vi "Get Request Type.vi"(8 "error in (no error)":errorcluster, 11 "GetStreamStatus in":refnum<class "GetStreamStatus.lvclass">) -> (0 "error out":errorcluster, 2 "Request Type":string, 3 "GetStreamStatus out":refnum<class "GetStreamStatus.lvclass">)   [LabVIEW 2022 SP3, in "obs-websocket-lv.lvlib" / "GetStreamStatus.lvclass"]
uses:
  GetStreamStatus.lvclass
  GetStreamStatus.lvclass/GetStreamStatus.ctl
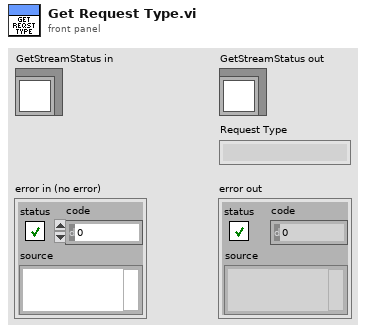
[diagram p1: front panel]
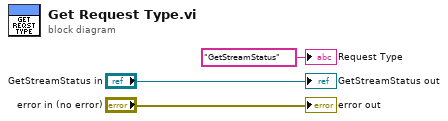
[diagram p0: block diagram]
diagram:
  "error out" <- "error in (no error)"
  "GetStreamStatus out" <- "GetStreamStatus in"
  "Request Type" <- "GetStreamStatus" ("Request Type")
